vi "Get value by Variant.vi"(8 "error in (no error)":errorcluster, 11 "Column in":refnum<class "Composed Column.lvclass">) -> (0 "error out":errorcluster, 2 "Variant":variant, 3 "Column out":refnum<class "Composed Column.lvclass">)   [LabVIEW 2020, in "Composed Columns.lvlib" / "Composed Column.lvclass"]
uses:
  Composed Column.lvclass
  Composed Column.lvclass/Composed Column.ctl
  Composed Columns/Value Source Interface Class/Value Source.lvclass
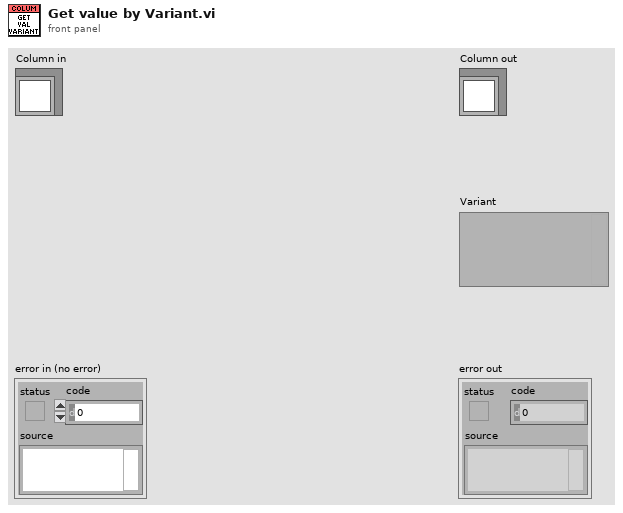
[diagram p1: front panel]
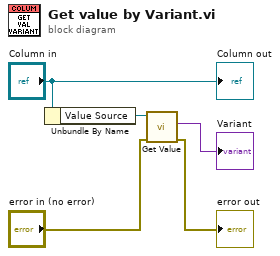
[diagram p0: block diagram]
diagram:
  n1 = Unbundle By Name("Column in") -> ("Value Source"=w5:refnum<class "Value Source.lvclass">)
  n2 = call-dynamic "Get Value.vi"("error in (no error)"="error in (no error)", "Value Source in"=w5) -> ("error out"=→"error out":errorcluster, "Value"=→"Variant":variant)  [unwired: 7 in, 1 out]
  "Column out" <- "Column in"
